vi "Vision Research Phantom Series PhCon PhGetCameraID.vi"(0 "CN in":u32=1, 5 "Error In (no error)":errorcluster) -> (14 "CN out":u32=1, 15 "pSerial":u32, 16 "pCameraName":string, 19 "Error Out":errorcluster)   [LabVIEW 2013, in "VRI.lvlib"]
doc: "PhCon.dll\n\nPhGetCameraID\nHRESULT PhGetCameraID(UINT CN, UINT *pSerial, char *pCameraName);\n\nParameters Description\nCN (in) Camera number.\npSerial (out) Factory serial.\npCameraName (out) Camera name maximum 15 char.\nReturn HRESULT (0=Ok)\nComments Get the serial number and/or the name of the camera.\n You can request only one information by setting the\n other parameter to NULL. The Serial number is set\n in the factory and it is unique for each camera while\n the camera name can be changed by the user.\n\nWritten by:\nBLOOMY CONTROLS, INC\nWINDSOR, CT 06095, USA\n860-298-9925\nwww.bloomy.com\nV1.0.0\nMay, 2004"
uses:
  VRI.lvlib
  Phantom DLLs/PhCon.dll
panel:
  # "For instructions on the use of this VI, press Ctrl+H to display the help window and move the mouse over the icon, controls, and indicators"
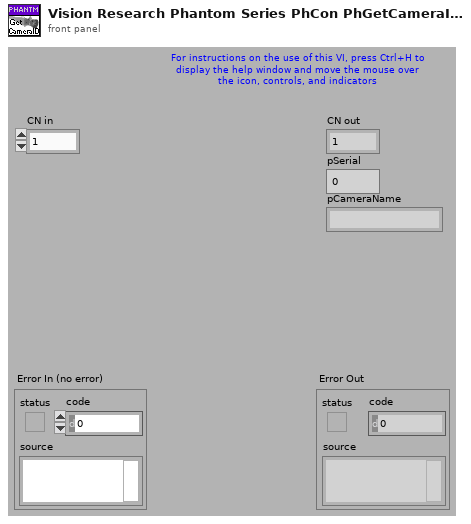
[diagram p1: front panel]
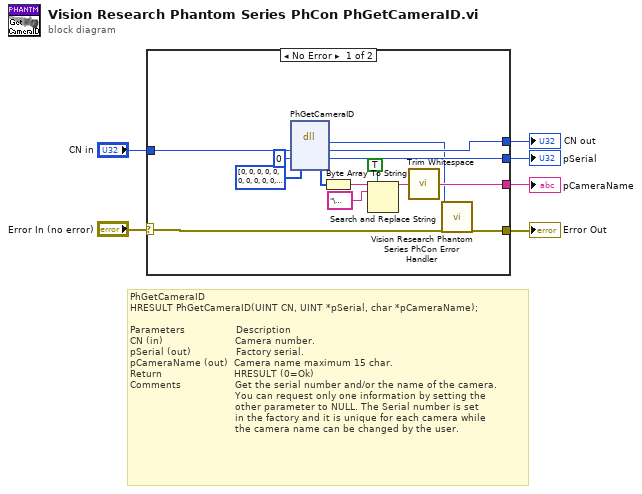
[diagram p0: block diagram]
diagram:
  # "PhGetCameraID\nHRESULT PhGetCameraID(UINT CN, UINT *pSerial, char *pCameraName);\n\nParameters                 Description\nCN (in)                        Camera number.\npSerial (out)               Factory serial.\npCameraName (out)  Camera name maximum 15 char.\nReturn                        HRESULT (0=Ok)\nComments                  Get the serial number and/or the name of the camera.\n                                   You can request only one information by setting the\n                                   other parameter to NULL. The Serial number is set\n                                   in the factory and it is unique for each camera while\n                                   the camera name can be changed by the user."
  n1 = case shown="No Error" "Error In (no error)" {
    selector: "Error In (no error)" -> [w20 w22]
    tunnel: [w19 w22] -> w5
    tunnel: "CN in" -> [w18 w21]
    tunnel: [w17 _] -> w3
    tunnel: [w16 _] -> w2
    tunnel: [w15 w21] -> w1
    frame No Error {
      n2 = dll-call lib="C:/Projects/SDK/32-bit/Vision Research Phantom Series Labview Driver/Phantom DLLs/PhCon.dll" fn="PhGetCameraID"("CN"=w18, "pSerial"=u32 0, "pCameraName"=u8[] [0, 0, 0, 0, 0, 0, 0, 0, 0, 0, 0, 0, 0, 0, 0]) -> ("HRESULT"=w14:i32, "CN"=w15:u32, "pSerial"=w17:u32, "pCameraName"=w12:u8[])  [unwired: 3 in, 2 out]
      n3 = Byte Array To String(unsigned byte array=w12) -> (string=w10:string)
      n4 = Search and Replace String(replace all?=TRUE ("replace all? (F)"), input string=w10, search string="\u0000") -> (result string=w9:string)  [unwired: 5 in, 3 out]
      n5 = call <vilib>:"Trim Whitespace.vi"("string"=w9) -> ("trimmed string"=w16:string)  [unwired: 1 in]
      n6 = call "Vision Research Phantom Series PhCon Error Handler.vi"("ErrNo"=w14, "Error In (no error)"=w20) -> ("Error Out"=w19:errorcluster)  [unwired: 17 out]
    }
    frame Error {
    }
  }
  "Error Out" <- w5
  "pSerial" <- w3
  "pCameraName" <- w2
  "CN out" <- w1
